vi "ToGraphVizString.vi"(9 "AST in":refnum<class "VI_Hierarchy.lvclass">) -> (3 "AST out":refnum<class "VI_Hierarchy.lvclass">, 4 "GraphViz string":string)   [LabVIEW 2014, in "VI_Hierarchy.lvclass"]
uses:
  VI_Hierarchy.lvclass
  VI_Hierarchy.lvclass/VI_Hierarchy.ctl
  DAG/DAG/DAG.lvclass/DAG.ctl
  DAG/DAG/DAG.lvclass
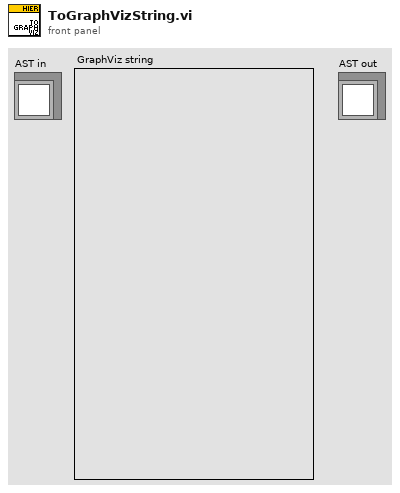
[diagram p1: front panel]
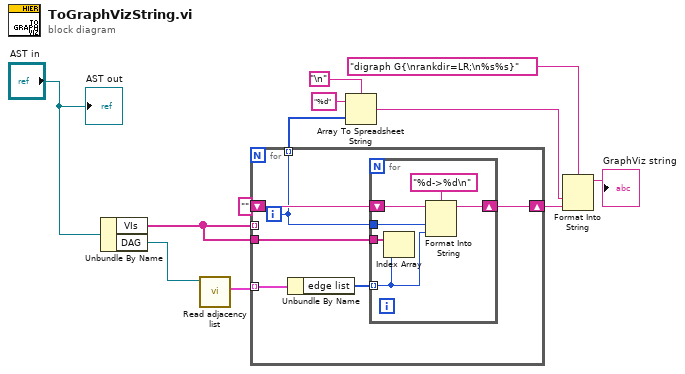
[diagram p0: block diagram]
diagram:
  n1 = Unbundle By Name("AST in") -> ("VIs"=w2:string[], "DAG"=w8:refnum<class "DAG.lvclass">)
  n2 = call "Read adjacency list.vi"("DAG in"=w8) -> ("adjacency list"=w7:cluster{"edge list":i32[]}[])  [unwired: 9 in, 1 out]
  n3 = for {
    tunnel: w7 -> [w18] mode=indexing
    shift-right: [w16] -> w10
    shift-left: "" -> [w15]
    tunnel: w2 -> [_] mode=indexing
    tunnel: w2 -> [w14]
    tunnel: [w13] -> w1 mode=indexing
    i -> [w13]
    n4 = Unbundle By Name(w18) -> ("edge list"=w17:i32[])
    n5 = for {
      tunnel: w17 -> [w19] mode=indexing
      tunnel: w13 -> [w21]
      shift-right: [w23] -> w16
      shift-left: w15 -> [w22]
      tunnel: w14 -> [w20]
      n6 = Index Array(array=w20, index=w19) -> ()  [unwired: 1 out]
      n7 = Format Into String(format string="%d->%d\n", initial string=w22, w21, w19) -> (resulting string=w23:string)  [unwired: 1 in, 1 out]
    }
  }
  n8 = Array To Spreadsheet String(delimiter (Tab)="\n", array=w1, 3:"%d" ("format string")) -> (spreadsheet string=w3:string)
  n9 = Format Into String(format string="digraph G{\nrankdir=LR;\n%s%s}", w3, w10) -> (resulting string=→"GraphViz string":string)  [unwired: 2 in, 1 out]
  "AST out" <- "AST in"
